vi "IMAQ Resample ROI.vi"(8 "Interp Ratio":dbl=2.5, 10 "Final Size":i32=400, 11 "Image In":T1=refnum) -> (3 "Image Out":T1)   [LabVIEW 2012, in "LightPipes.lvlib"]
uses:
  LightPipes.lvlib
  <vilib>/vision/Image Controls.llb/IMAQ Image.ctl
  <vilib>/vision/NI_Vision_Development_Module.lvlib
panel:
  out "Optional Rectangle":u32[](array[numeric])
  out "Num Row":i32=480
  out "Num Col":i32=640
  out "Centroid":cluster{"X Centroid":sgl, "Y Centroid":sgl}={"X Centroid"=430.19534, "Y Centroid"=287.30713} {"Y Centroid" format="%.2f"; "X Centroid" format="%.2f"}
  out "Image":T1(plugin-control)
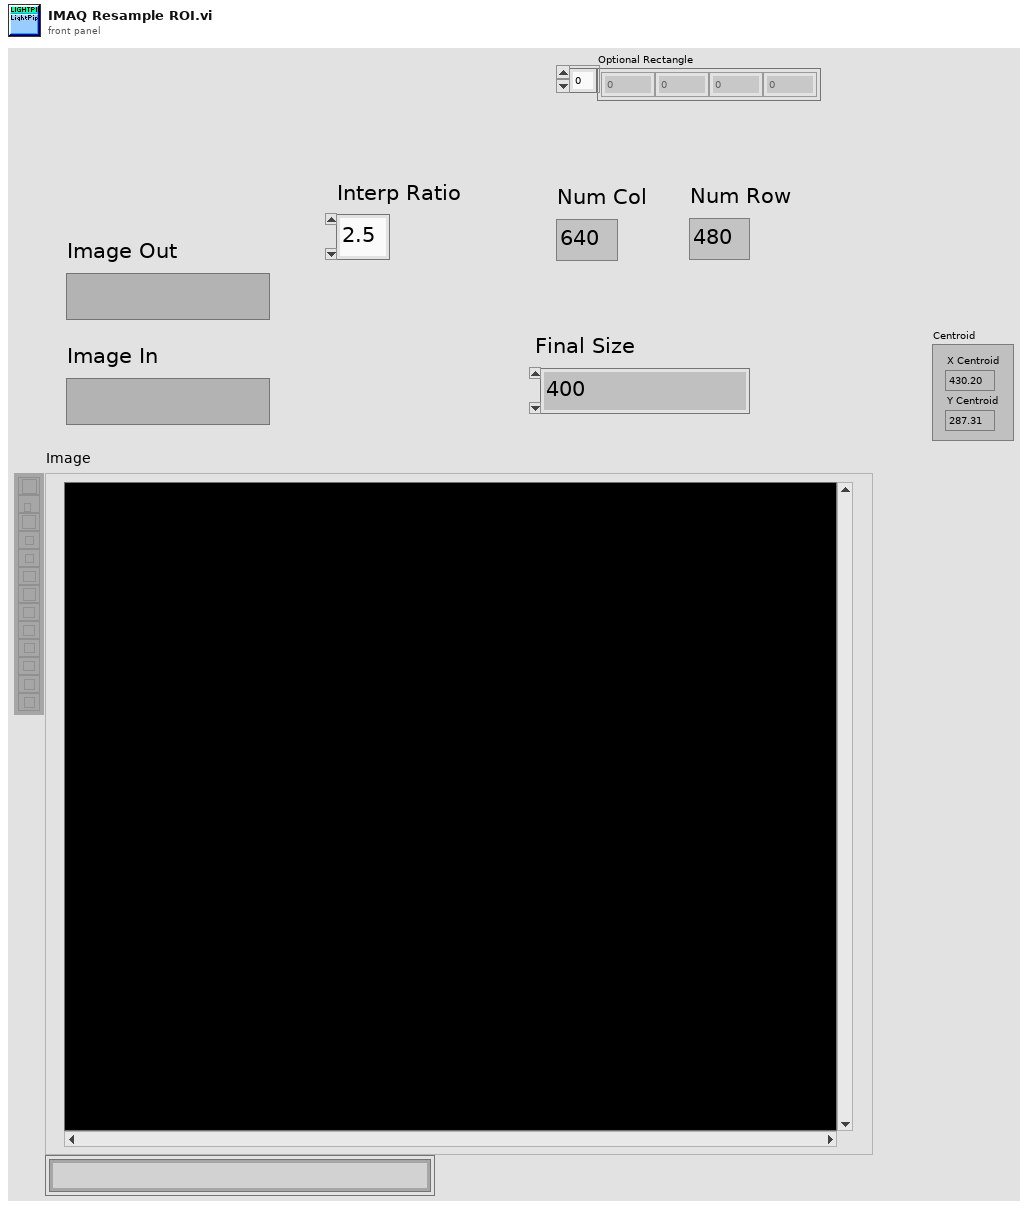
[diagram p1: front panel]
types:
  T1 = typedef "IMAQ Image.ctl" = refnum<image>
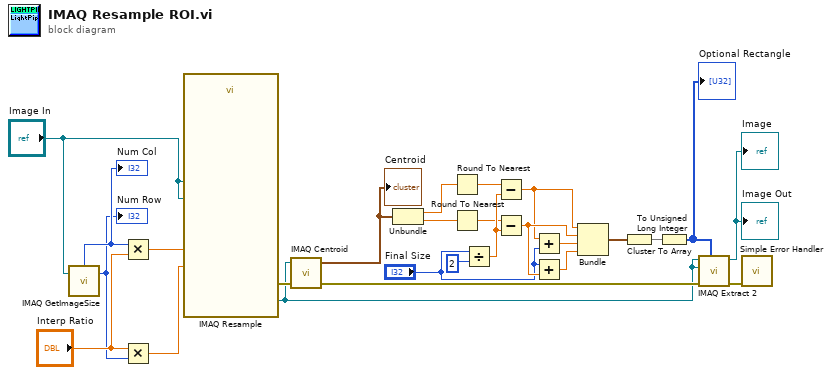
[diagram p0: block diagram]
diagram:
  n1 = call "IMAQ GetImageSize"("Image"="Image In") -> ("Y Resolution"=w10:i32, "X Resolution"=w13:i32)  [unwired: 3 in, 1 out]
  "Num Col" <- w13
  "Num Row" <- w10
  n2 = Multiply(x=w13, y="Interp Ratio") -> (x*y=w12:dbl)
  n3 = Multiply(x="Interp Ratio", y=w10) -> (x*y=w9:dbl)
  n4 = call "IMAQ Resample"("X Resolution"=w12, "Y Resolution"=w9, "Image Dst"="Image In", "Image Src"="Image In") -> ("error out"=w7:errorcluster, "Image Dst Out"=w2:T1)  [unwired: 6 in]
  n5 = call "IMAQ Centroid"("error in (no error)"=w7, "Image"=w2) -> ("error out"=w6:errorcluster, "Centroid"=w26:cluster{"X Centroid":sgl, "Y Centroid":sgl})  [unwired: 2 in]
  "Centroid" <- w26
  n6 = Unbundle(w26) -> ("X Centroid"=w25:sgl, "Y Centroid"=w24:sgl)
  n7 = Round To Nearest(number=w25) -> (nearest integer value=w19:sgl)
  n8 = Round To Nearest(number=w24) -> (nearest integer value=w18:sgl)
  n9 = Divide(x="Final Size", y=2) -> (x/y=w20:dbl)
  n10 = Subtract(x=w19, y=w20) -> (x-y=w22:dbl)
  n11 = Subtract(x=w18, y=w20) -> (x-y=w23:dbl)
  n12 = Add(x=w22, y="Final Size") -> (x+y=w16:dbl)
  n13 = Add(x="Final Size", y=w23) -> (x+y=w15:dbl)
  n14 = Bundle "Bundle"(w22, w23, w16, w15) -> (w17:cluster{dbl, dbl, dbl, dbl})  [unwired: 1 in]
  n15 = Cluster To Array(cluster=w17) -> (array=w4:dbl[])
  n16 = To Unsigned Long Integer(number=w4) -> (unsigned 32bit integer=w1:u32[])
  "Optional Rectangle" <- w1
  n17 = call "IMAQ Extract 2"("Optional Rectangle"=w1, "error in (no error)"=w6, "Image Dst"=w2, "Image Src"=w2) -> ("error out"=w5:errorcluster, "Image Dst Out"=→"Image" →"Image Out":T1)  [unwired: 6 in]
  n18 = call <vilib>:"Simple Error Handler.vi"("error in (no error)"=w5) -> ()  [unwired: 4 in, 5 out]
